vi "Check Firmware Compatibility.vi"(8 "error in (no error)":errorcluster, 11 "TD in":refnum<class "Test Device.lvclass">) -> (0 "error out":errorcluster, 3 "TD out":refnum<class "Test Device.lvclass">)   [LabVIEW 2015, in "Test Device.lvclass"]
uses:
  Test Device.lvclass
  Test Device.lvclass/Test Device.ctl
  <vilib>/plasmapper/PL BlackBox Modbus CLient/PL BlackBox Modbus Client.lvclass
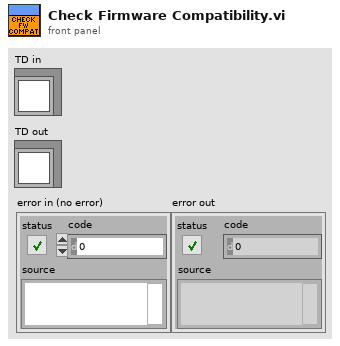
[diagram p1: front panel]
types:
  T1 = cluster{"hardware":cluster{"name":string, "version":cluster{"major":u16, "minor":u16, "patch":u16}, "uid":string}, "firmware":cluster{"name":string, "version":cluster{"major":u16, "minor":u16, "patch":u16}}, "number of hardware interfaces":u16, "number of servers":u16}
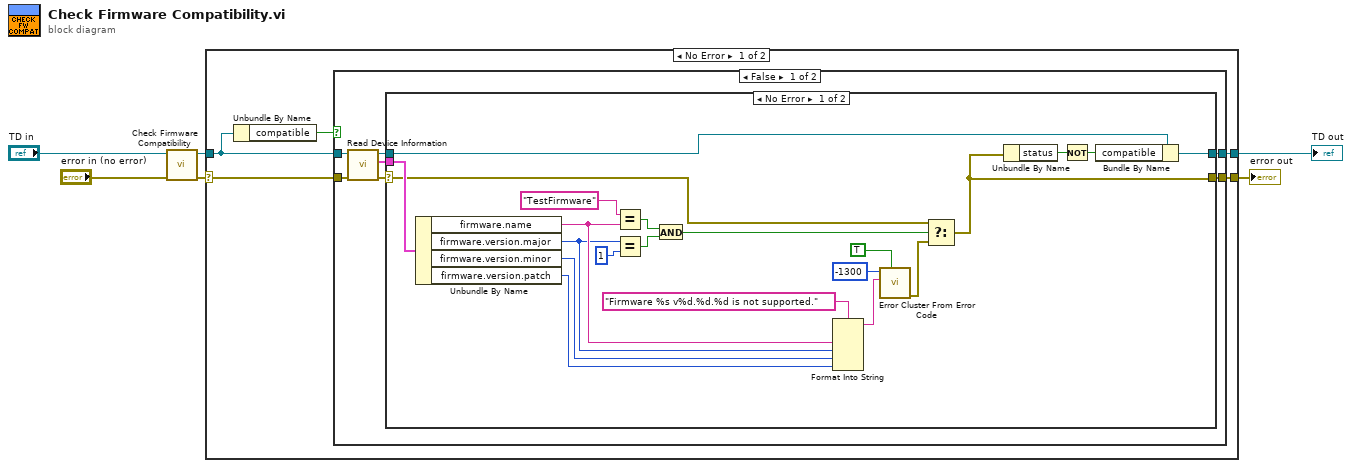
[diagram p0: block diagram]
diagram:
  n1 = call-parent "Check Firmware Compatibility.vi"("error in (no error)"="error in (no error)", "PLBB in"="TD in") -> ("error out"=w1:errorcluster, "PLBB out"=w4:refnum<class "Test Device.lvclass">)  [unwired: 8 in]
  n2 = case shown="No Error" w1 {
    selector: w1 -> [w9 w45]
    tunnel: w4 -> [w8 w44]
    tunnel: [w11 w44] -> w3
    tunnel: [w10 w45] -> w2
    frame No Error {
      n3 = Unbundle By Name(w8) -> ("compatible"=w7:bool)
      n4 = case shown="False" w7 {
        tunnel: [w15 w43] -> w11
        tunnel: [w14 w42] -> w10
        tunnel: w9 -> [w13 w42]
        tunnel: w8 -> [w12 w43]
        frame False {
          n5 = call <vilib>:"Read Device Information.vi"("error in (no error)"=w13, "PLBB in"=w12) -> ("error out"=w18:errorcluster, "device information"=w16:T1, "PLBB out"=w17:refnum<class "Test Device.lvclass">)  [unwired: 7 in]
          n6 = case shown="No Error" w18 {
            selector: w18 -> [w33 w40]
            tunnel: w17 -> [w21 w41]
            tunnel: w16 -> [w39 _]
            tunnel: [w20 w41] -> w15
            tunnel: [w19 w40] -> w14
            frame No Error {
              n7 = Unbundle By Name(w39) -> ("firmware.name"=w27:string, "firmware.version.major"=w26:u16, "firmware.version.minor"=w25:u16, "firmware.version.patch"=w24:u16)
              n8 = Equal?(x="TestFirmware", y=w27) -> (x = y?=w36:bool)
              n9 = Equal?(x=w26, y=u16 1) -> (x = y?=w35:bool)
              n10 = And(x=w36, y=w35) -> (x .and. y?=w34:bool)
              n11 = Format Into String(format string="Firmware %s v%d.%d.%d is not supported." ("error message (\"\")"), w27, w26, w25, w24) -> (resulting string=w32:string)  [unwired: 2 in, 1 out]
              n12 = call <vilib>:"Error Cluster From Error Code.vi"("show call chain? (False)"=TRUE, "error message (\"\")"=w32, "error code (0)"=-1300) -> ("error out"=w28:errorcluster)  [unwired: 6 in]
              n13 = Select(t=w33, s=w34, f=w28) -> (s? t:f=w19:errorcluster)
              n14 = Unbundle By Name(w19) -> ("status"=w23:bool)
              n15 = Not(x=w23) -> (.not. x?=w22:bool)
              n16 = Bundle By Name(cluster=w21, "compatible"=w22) -> (w20:refnum<class "Test Device.lvclass">)
            }
            frame Error {
            }
          }
        }
        frame True {
        }
      }
    }
    frame Error {
    }
  }
  "error out" <- w2
  "TD out" <- w3
